vi "Limelight Record Values.vi"(0 "tv":dbl, 5 "Steer":dbl, 7 "tx":dbl, 9 "ta":dbl, 11 "Drive":dbl) -> ()   [LabVIEW 2020]
uses:
  <vilib>/Analysis/Matrix/Numeric/Conversions/Matrix To Array - RM.vi
  Framework/Robot Global Data.vi
  <vilib>/Utility/file.llb/Write Delimited Spreadsheet (DBL).vi
  <vilib>/Analysis/Matrix/NI_Matrix.lvlib
panel:
  in  "Record Path":bool
  out "path":path
  out "error out":errorcluster
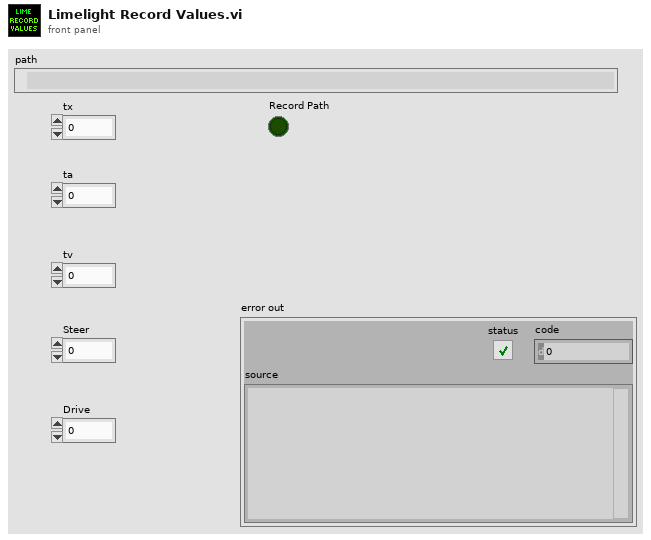
[diagram p1: front panel]
types:
  T1 = typedef "NI_Matrix.lvlib/RealMatrix.ctl" = dbl[][]
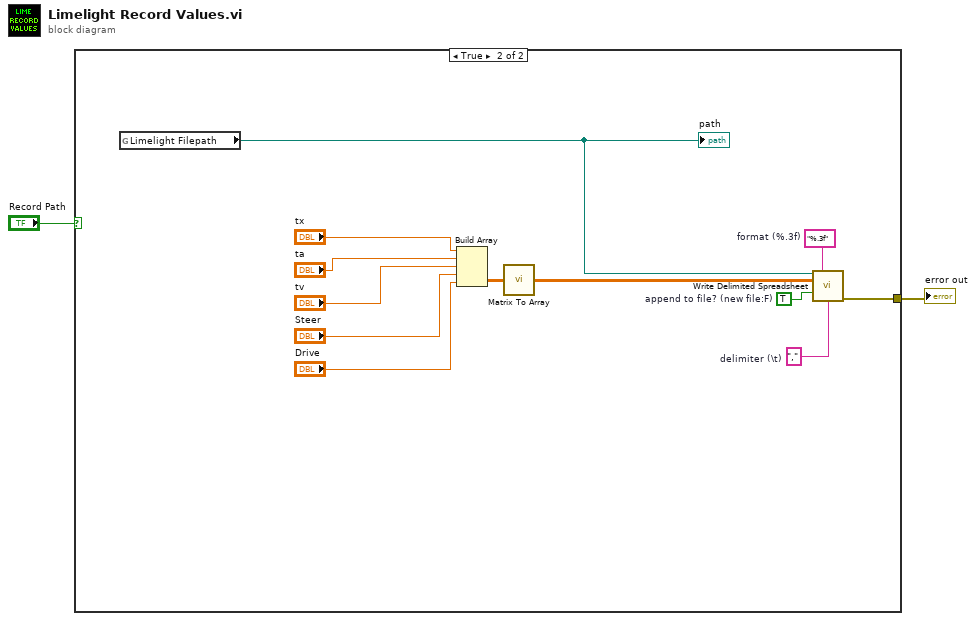
[diagram p0: block diagram]
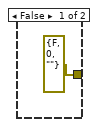
[diagram p2: hidden frame]
diagram:
  n1 = case shown="True" "Record Path" {
    tunnel: [errorcluster {"status"=FALSE, "code"=0, "source"=""} ("error out") w13] -> w2
    frame False {
    }
    frame True {
      w11 = TRUE  # append to file? (new file:F)
      w12 = "%.3f"  # format (%.3f)
      w10 = ","  # delimiter (\t)
      n2 = global read "Robot Global Data.vi" "Limelight Filepath"() -> (w9:path)
      "path" <- w9
      n3 = Build Array("tx", "ta", "tv", "Steer", "Drive") -> (w15:T1)
      n4 = call-poly <vilib>:"Matrix To Array.vi"("Real Matrix"=w15) -> ("Real 2D Array"=w14:dbl[][])
      n5 = call-poly <vilib>:"Write Delimited Spreadsheet.vi"("file path (dialog if empty)"=w9, "format (%.3f)"=w12, "2D data"=w14, "append to file? (new file:F)"=w11, "delimiter (\\t)"=w10) -> ("error out"=w13:errorcluster)  [unwired: 9 in, 1 out]
    }
  }
  "error out" <- w2
